vi "Sonar.vi"(7 "Action":T4=enum."ReadValue", 8 "error in (no error)":errorcluster, 9 "Scaling factor (V/in)":dbl=0.009585, 11 "AIDeviceRef":T1={"DevStatus"={"status"=FALSE, "code"=0, "source"=""}, "Analog Module"=enum."Analog Module 1", "Analog Channel"=enum."Invalid"}) -> (0 "error out":errorcluster, 2 "distance":dbl(slide)=255.4405658841941 scale=0.0..250.0 scale format="%3d")   [LabVIEW 2013]
doc: "This example shows how to use the MaxBotix LV-MaxSonar-EZ1 Sonar Range Finder MB1010. It will display the distance from the sensor in inches.\n\nThis example works with the NI 9201 module with an Analog Breakout attached. The Analog Breakout should have 12V applied to the WAGO connector (J3). The sensor is attached to the 3x8 header using a 3-pin PWM connector."
uses:
  SonarAction.ctl
  <vilib>/Rock Robotics/WPI/AnalogChannel/WPI_AnalogChannelDevRef.ctl
  <vilib>/Rock Robotics/SystemInterfaces/Typedef/FPGA_TypedefAnalogModule.ctl
  <vilib>/Rock Robotics/SystemInterfaces/AI/FPGA_AIChannel.ctl
panel:
  in  "Average Bits":u8=3
  in  "Samples Per Second":dbl=1000.0
  # "Output information."
  # "EZ1"
  # "inches"
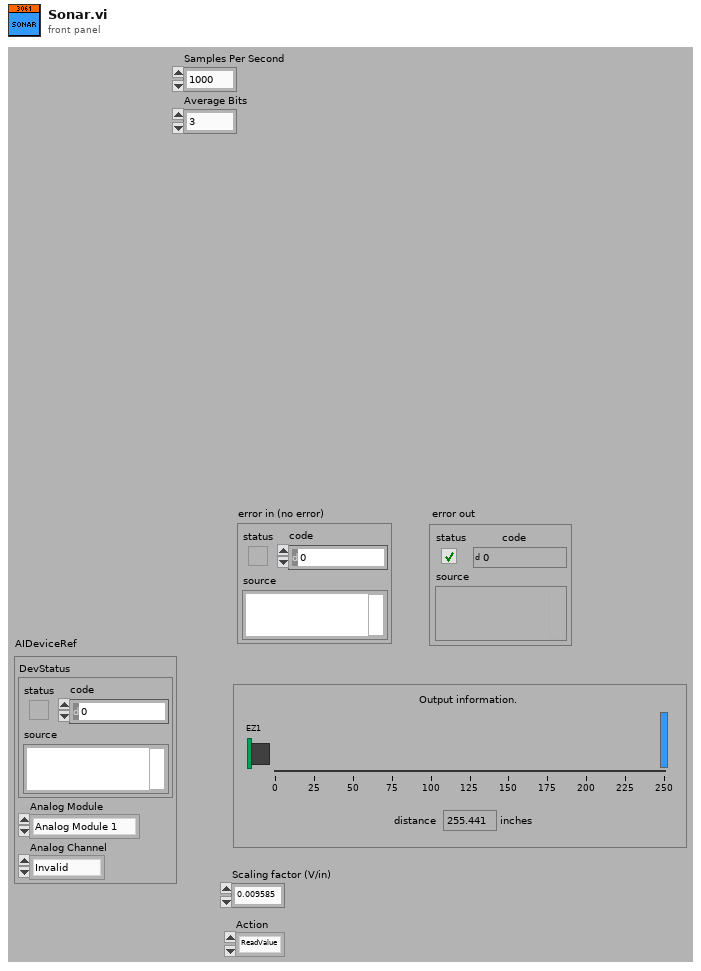
[diagram p1: front panel]
types:
  T1 = typedef "WPI_AnalogChannelDevRef.ctl" = cluster{"DevStatus":errorcluster, "Analog Module":T2, "Analog Channel":T3}
  T2 = typedef "FPGA_TypedefAnalogModule.ctl" = enum16{"Analog Module 1", "Analog Module 2"}
  T3 = typedef "FPGA_AIChannel.ctl" = enum8{"AI 1", "AI 2", "AI 3", "AI 4", "AI 5", "AI 6", "AI 7", "AI 8", "Invalid"}
  T4 = typedef "SonarAction.ctl" = enum16{"Init", "ReadValue", "Disable"}
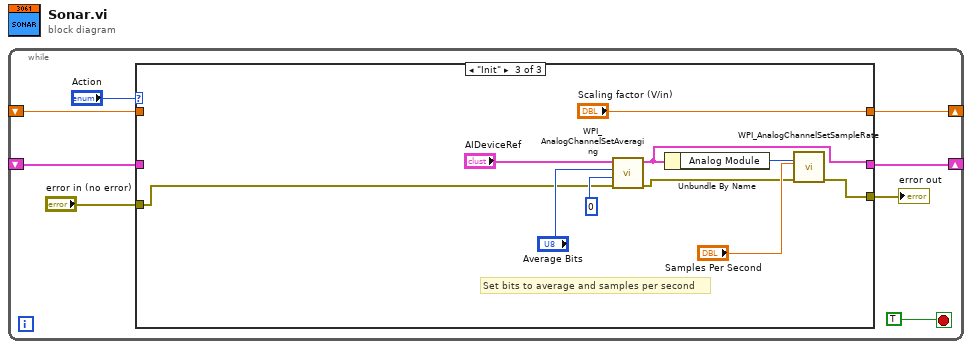
[diagram p0: block diagram]
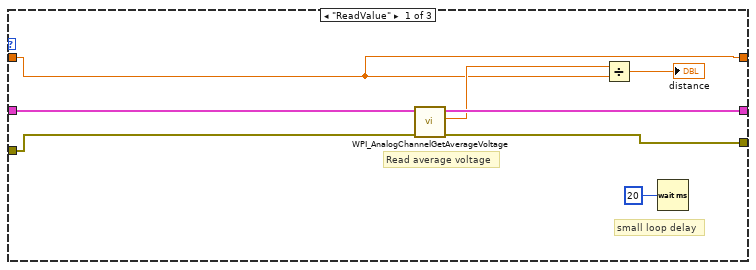
[diagram p2: hidden frame]
diagram:
  n1 = while {
    shift-right: [w5] -> _
    shift-left: _ -> [w8]
    shift-right: [w2] -> _
    shift-left: _ -> [w1]
    stop <- TRUE stop-if-true
    n2 = case shown="\"Init\"" "Action" {
      tunnel: [w16 w19 w24] -> w5
      tunnel: w8 -> [w11 w19 _]
      tunnel: [w10 w18 w23] -> w3
      tunnel: "error in (no error)" -> [w12 w18 w21]
      tunnel: [w9 w17 "Scaling factor (V/in)"] -> w2
      tunnel: w1 -> [w9 w17 _]
      frame "ReadValue" {
        # "small loop delay"
        # "Read average voltage"
        n3 = call <vilib>:"WPI_AnalogChannelGetAverageVoltage.vi"("error in (no error)"=w12, "AIDeviceRef"=w11) -> ("error out"=w10:errorcluster, "Voltage"=w14:dbl, "AIDeviceRef"=w16:T1)  [unwired: 7 out]
        n4 = Divide(x=w14, y=w9) -> (x/y=→"distance":dbl)
        n5 = Wait (ms)(milliseconds to wait=u32 20) -> ()  [unwired: 1 out]
      }
      frame "Disable" {
      }
      frame "Init" {
        # "Set bits to average and samples per second"
        n6 = call <vilib>:"WPI_AnalogChannelSetAveraging.vi"("error in (no error)"=w21, "OversampleBits"=u8 0, "AverageBits"="Average Bits", "AIDeviceRef"="AIDeviceRef") -> ("error out"=w25:errorcluster, "AIDeviceRef"=w24:T1)  [unwired: 6 out]
        n7 = Unbundle By Name(w24) -> ("Analog Module"=w26:T2)
        n8 = call <vilib>:"WPI_AnalogChannelSetSampleRate.vi"("error in (no error)"=w25, "Samples Per Second"="Samples Per Second", "Analog Module (Module 1)"=w26) -> ("error out"=w23:errorcluster)  [unwired: 1 in, 7 out]
      }
    }
    "error out" <- w3
  }
